vi "ReadDataFromBeckhoff.vi"(6 "error in (no error)":errorcluster, 8 "ReadGrpSymbols":string[](array[string]), 9 "Handle In":u32 format="%x") -> (0 "error out":errorcluster, 1 "BeckhoffParameters":T3, 2 "BeckhoffParamsRawData":T1, 3 "Handle Out":u32)   [LabVIEW 2020]
uses:
  <userlib>/Beckhoff-LabVIEW-Interface/_DependsOn/With TypeResolving/Read Sync Single TypeResolved.vi
panel:
  out "BeckhoffParamReadStatus":T2
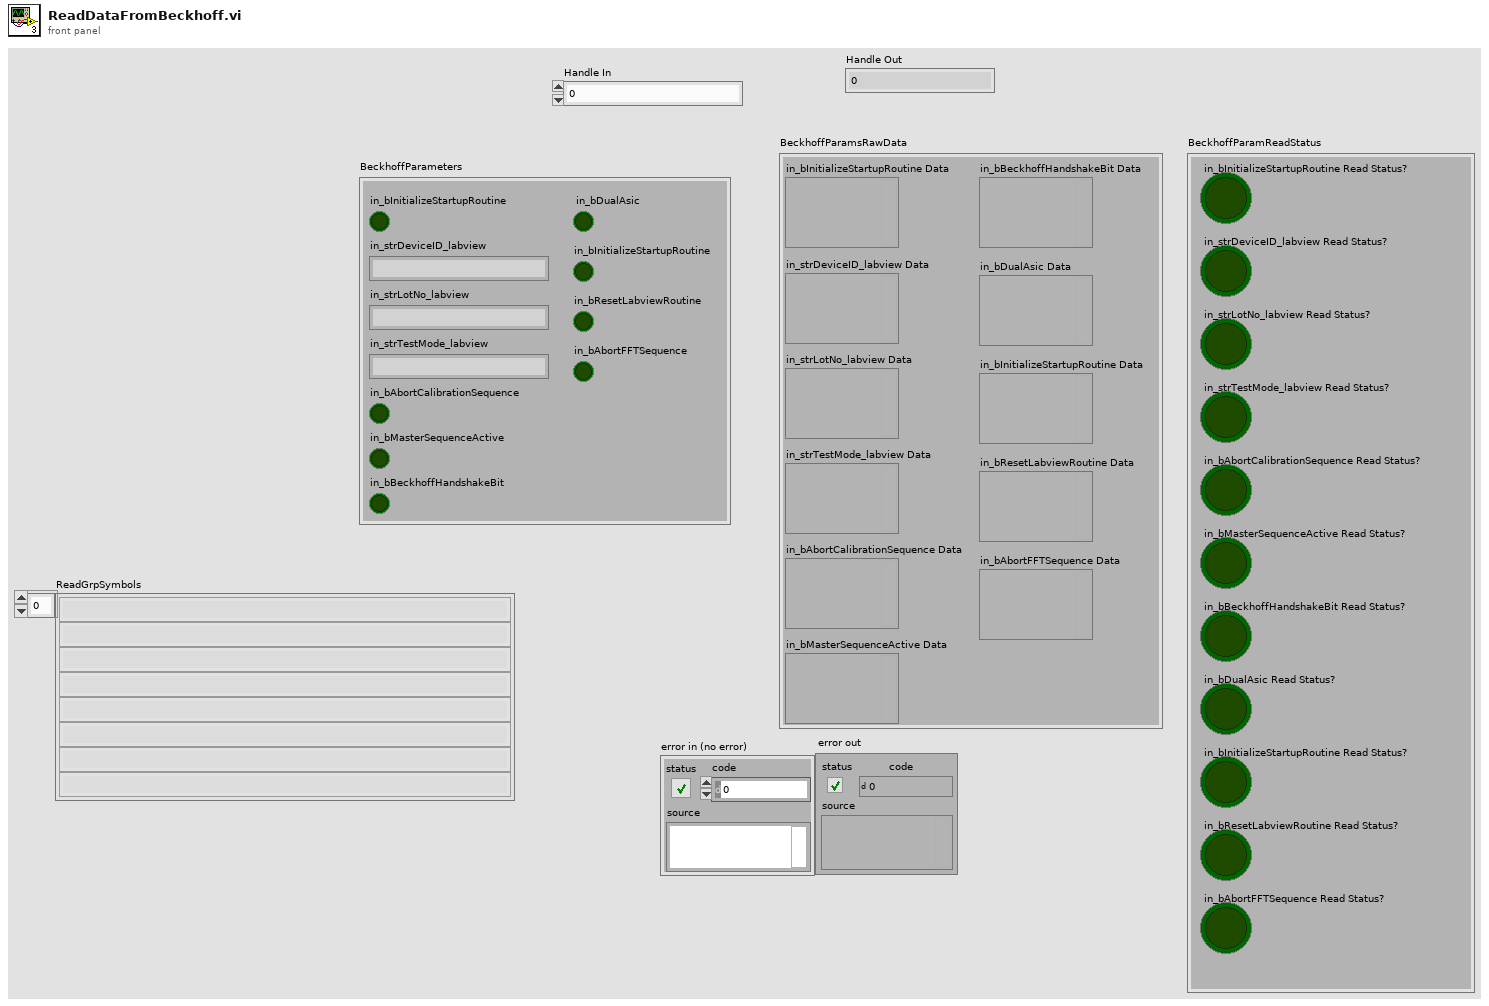
[diagram p1: front panel]
types:
  T1 = cluster{"in_bInitializeStartupRoutine Data":variant, "in_strDeviceID_labview Data":variant, "in_strLotNo_labview Data":variant, "in_strTestMode_labview Data":variant, "in_bAbortCalibrationSequence Data":variant, "in_bMasterSequenceActive Data":variant, "in_bBeckhoffHandshakeBit Data":variant, "in_bDualAsic Data":variant, "in_bInitializeStartupRoutine Data":variant, "in_bResetLabviewRoutine Data":variant, "in_bAbortFFTSequence Data":variant}
  T2 = cluster{"in_bInitializeStartupRoutine Read Status?":bool, "in_strDeviceID_labview Read Status?":bool, "in_strLotNo_labview Read Status?":bool, "in_strTestMode_labview Read Status?":bool, "in_bAbortCalibrationSequence Read Status?":bool, "in_bMasterSequenceActive Read Status?":bool, "in_bBeckhoffHandshakeBit Read Status?":bool, "in_bDualAsic Read Status?":bool, "in_bInitializeStartupRoutine Read Status?":bool, "in_bResetLabviewRoutine Read Status?":bool, "in_bAbortFFTSequence Read Status?":bool}
  T3 = cluster{"in_bInitializeStartupRoutine":bool, "in_strDeviceID_labview":string, "in_strLotNo_labview":string, "in_strTestMode_labview":string, "in_bAbortCalibrationSequence":bool, "in_bMasterSequenceActive":bool, "in_bBeckhoffHandshakeBit":bool, "in_bDualAsic":bool, "in_bInitializeStartupRoutine":bool, "in_bResetLabviewRoutine":bool, "in_bAbortFFTSequence":bool}
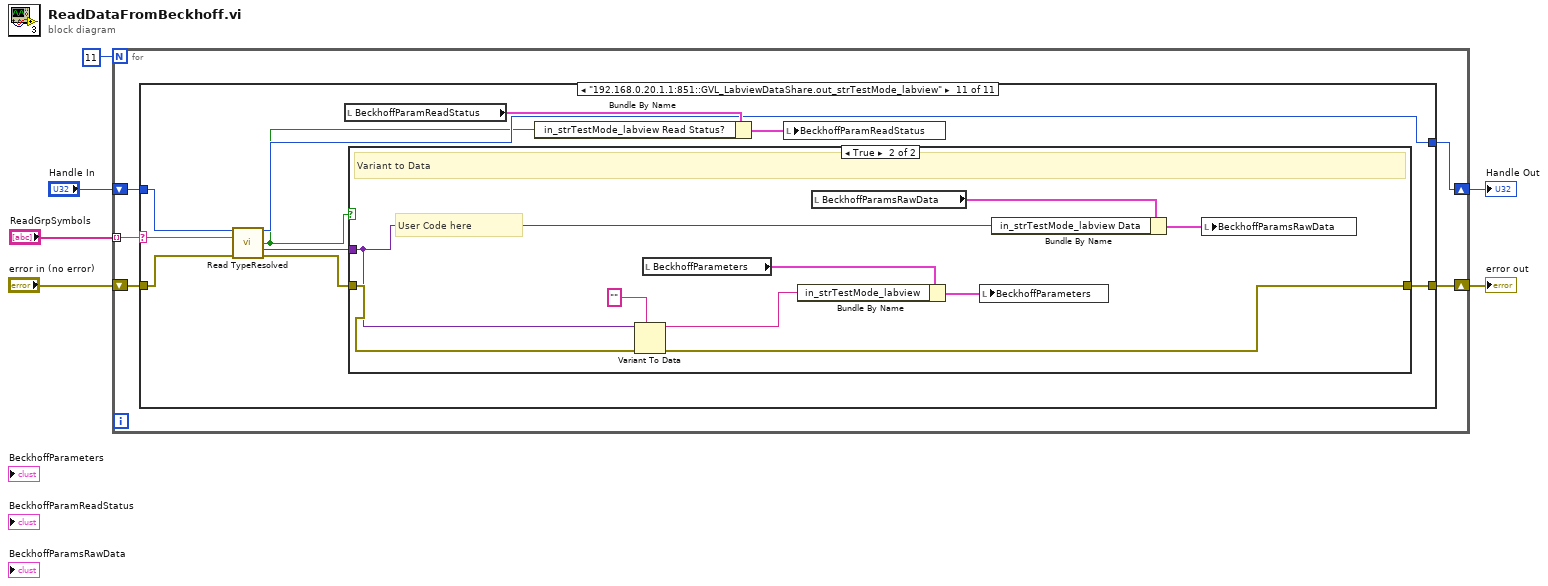
[diagram p0: block diagram]
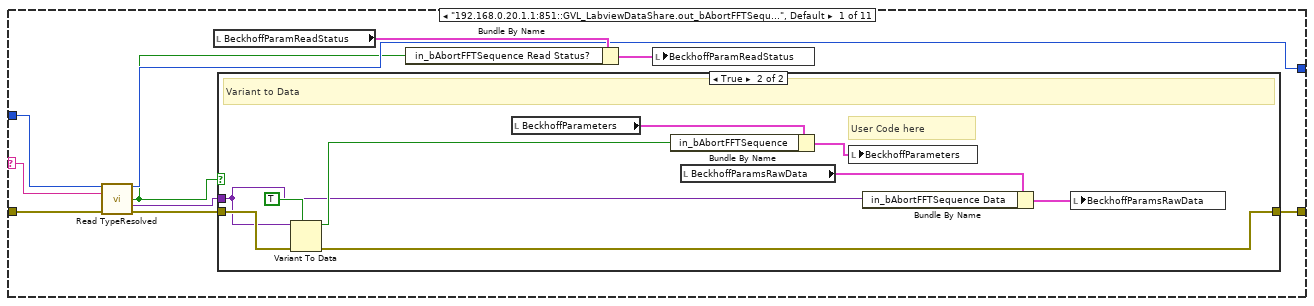
[diagram p2: hidden frame]
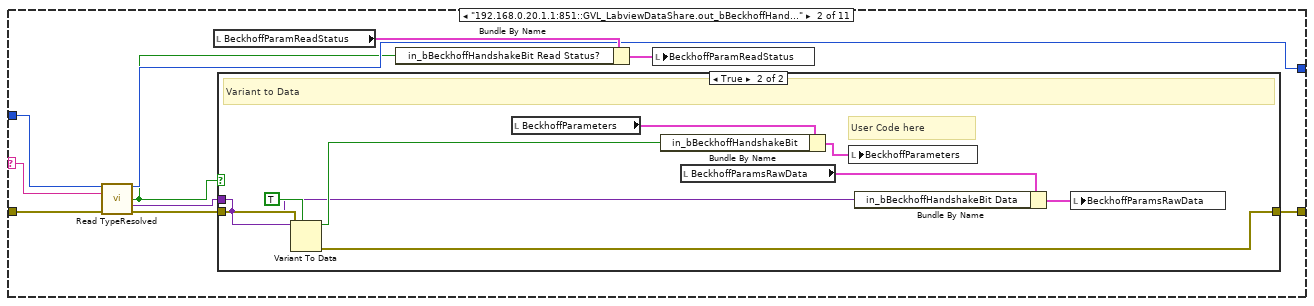
[diagram p4: hidden frame]
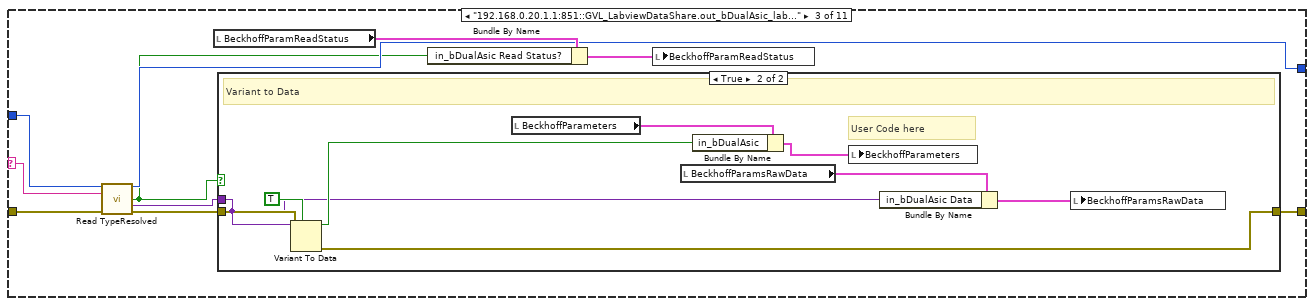
[diagram p6: hidden frame]
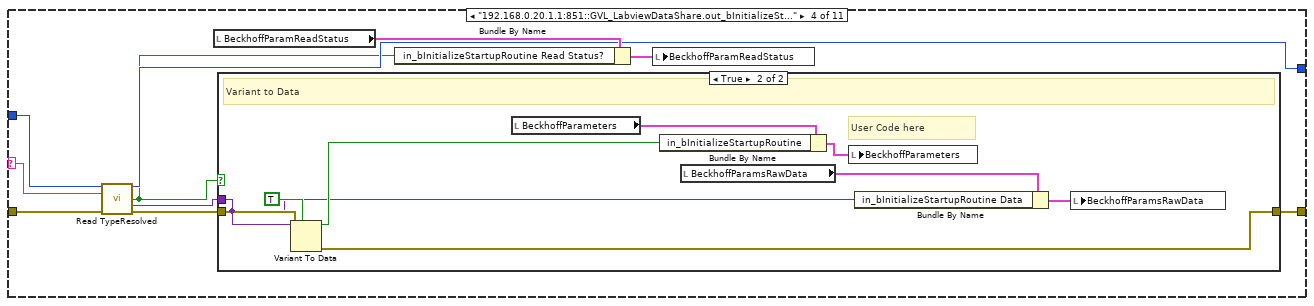
[diagram p8: hidden frame]
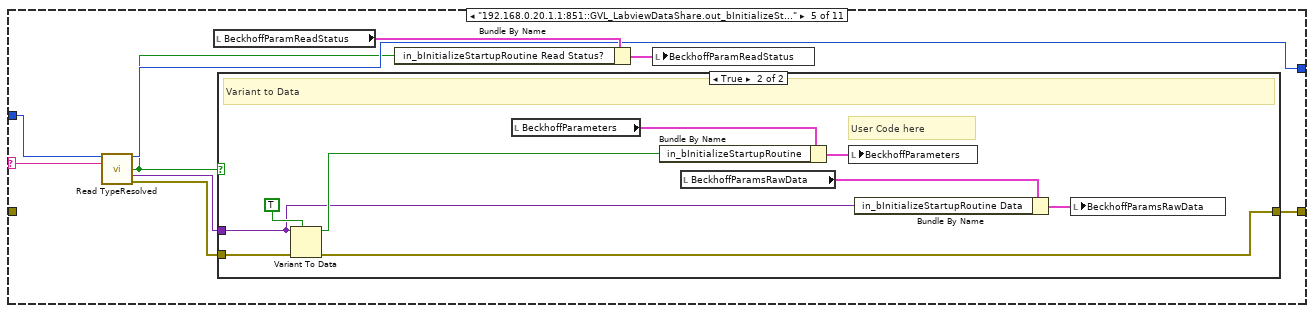
[diagram p10: hidden frame]
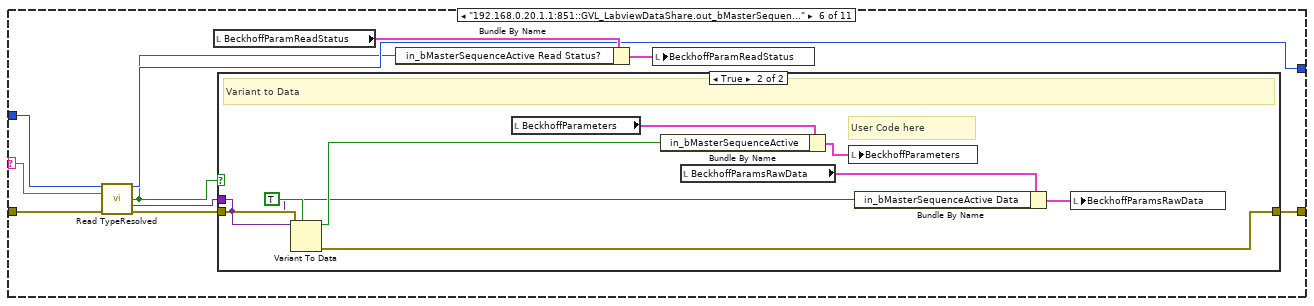
[diagram p12: hidden frame]
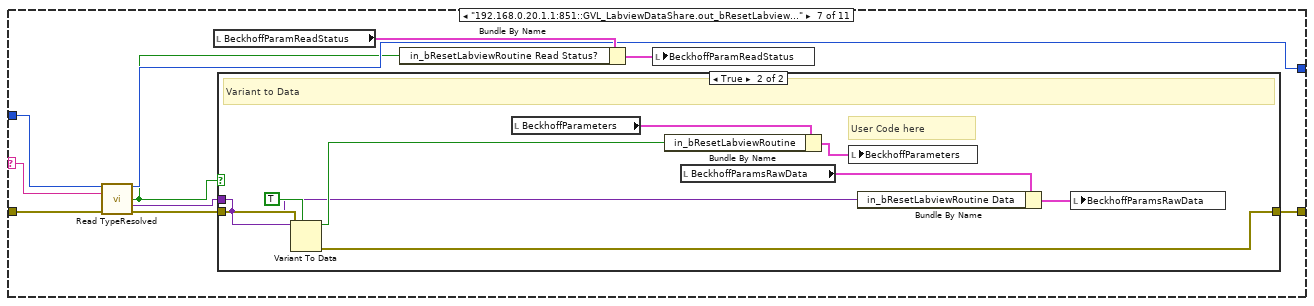
[diagram p14: hidden frame]
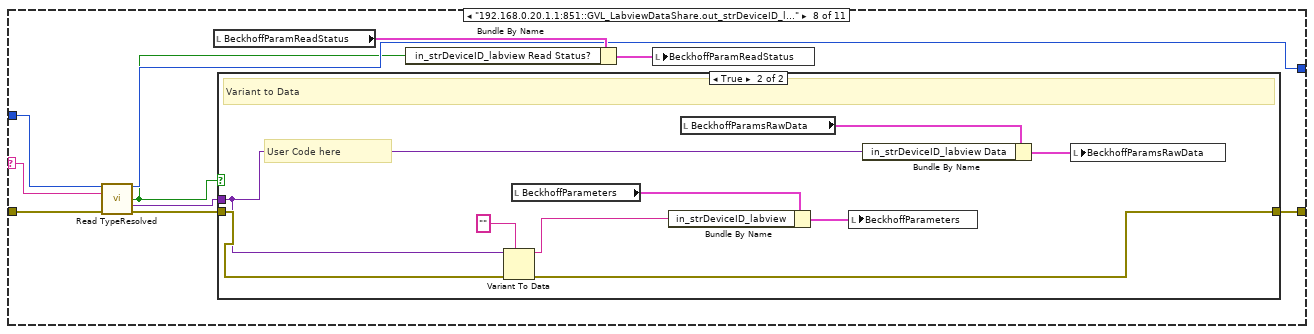
[diagram p16: hidden frame]
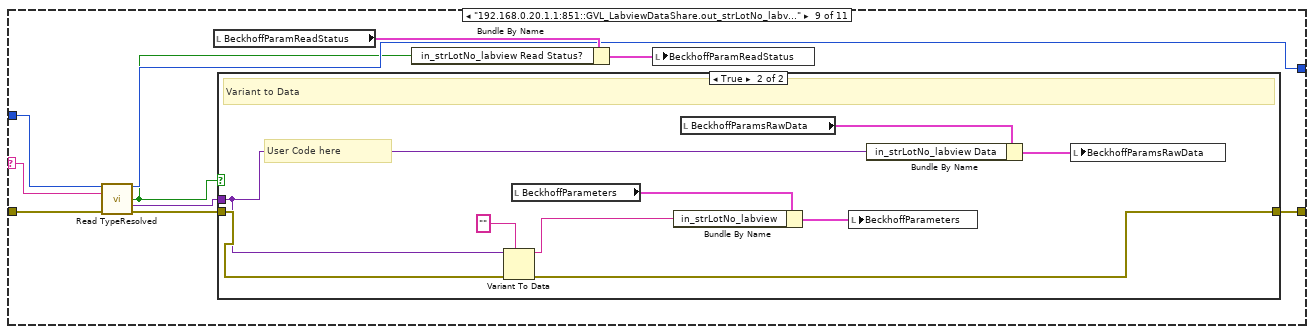
[diagram p18: hidden frame]
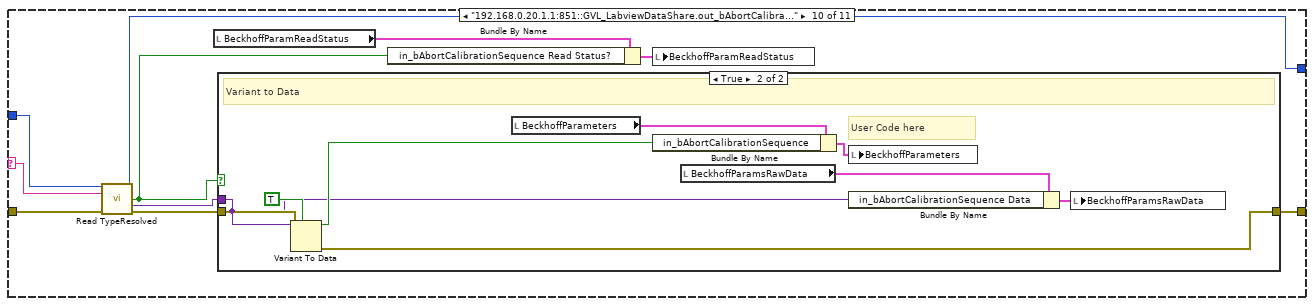
[diagram p20: hidden frame]
diagram:
  n1 = for {
    N: 11 -> [_]
    tunnel: "ReadGrpSymbols" -> [w11] mode=indexing
    shift-right: [w9] -> w2
    shift-left: "error in (no error)" -> [w10]
    shift-right: [w7] -> w1
    shift-left: "Handle In" -> [w8]
    n2 = case shown="\"192.168.0.20.1.1:851::GVL_LabviewDataShare.out_strTestMode_labview\"" w11 {
      selector: w11 -> [w15 w34 w54 w74 w96 w114 w135 w154 w174 w197 w214]
      tunnel: w10 -> [w16 w36 w55 w75 _ w115 w136 w155 w175 w200 w215]
      tunnel: [w13 w37 w57 w77 w93 w116 w132 w156 w176 w193 w216] -> w9
      tunnel: w8 -> [w17 w35 w56 w76 w95 w113 w134 w153 w173 w199 w213]
      tunnel: [w14 w33 w53 w73 w94 w112 w133 w152 w172 w198 w212] -> w7
      frame "192.168.0.20.1.1:851::GVL_LabviewDataShare.out_bAbortFFTSequence_labview", Default {
        n3 = call-poly <userlib>:"Read TypeResolved.vi"("Handle"=w17, "SymbolName"=w15, "error constant"=w16) -> ("Handle"=w14:u32, "Read Status?"=w12:bool, "RData"=w18:variant, "error out"=w19:errorcluster)  [unwired: 9 in]
        n4 = local read "BeckhoffParamReadStatus"() -> (w21:T2)
        n5 = case shown="True" w12 {
          tunnel: w19 -> [w22 w31]
          tunnel: [w22 w30] -> w13
          tunnel: w18 -> [_ w23]
          frame False {
            # "Read Data failed"
            # "Read Status"
          }
          frame True {
            # "User Code here"
            # "Variant to Data"
            n6 = Variant To Data(error in=w31, type=TRUE, Variant=w23) -> (data=w26:bool, error out=w30:errorcluster)
            n7 = local read "BeckhoffParameters"() -> (w28:T3)
            n8 = Bundle By Name(cluster=w28, "in_bAbortFFTSequence"=w26) -> (w27:T3)
            n9 = local read "BeckhoffParamsRawData"() -> (w25:T1)
            n10 = local write "BeckhoffParameters"(w27) -> ()
            n11 = Bundle By Name(cluster=w25, "in_bAbortFFTSequence Data"=w23) -> (w24:T1)
            n12 = local write "BeckhoffParamsRawData"(w24) -> ()
          }
        }
        n13 = Bundle By Name(cluster=w21, "in_bAbortFFTSequence Read Status?"=w12) -> (w20:T2)
        n14 = local write "BeckhoffParamReadStatus"(w20) -> ()
      }
      frame "192.168.0.20.1.1:851::GVL_LabviewDataShare.out_bBeckhoffHandshakeBit_labview" {
        n15 = call-poly <userlib>:"Read TypeResolved.vi"("Handle"=w35, "SymbolName"=w34, "error constant"=w36) -> ("Handle"=w33:u32, "Read Status?"=w32:bool, "RData"=w38:variant, "error out"=w39:errorcluster)  [unwired: 9 in]
        n16 = local read "BeckhoffParamReadStatus"() -> (w41:T2)
        n17 = case shown="True" w32 {
          tunnel: w39 -> [w42 w51]
          tunnel: [w42 w50] -> w37
          tunnel: w38 -> [_ w43]
          frame False {
            # "Read Data failed"
            # "Read Status"
          }
          frame True {
            # "User Code here"
            # "Variant to Data"
            n18 = Variant To Data(error in=w51, type=TRUE, Variant=w43) -> (data=w46:bool, error out=w50:errorcluster)
            n19 = local read "BeckhoffParameters"() -> (w48:T3)
            n20 = Bundle By Name(cluster=w48, "in_bBeckhoffHandshakeBit"=w46) -> (w47:T3)
            n21 = local read "BeckhoffParamsRawData"() -> (w44:T1)
            n22 = local write "BeckhoffParameters"(w47) -> ()
            n23 = Bundle By Name(cluster=w44, "in_bBeckhoffHandshakeBit Data"=w43) -> (w45:T1)
            n24 = local write "BeckhoffParamsRawData"(w45) -> ()
          }
        }
        n25 = Bundle By Name(cluster=w41, "in_bBeckhoffHandshakeBit Read Status?"=w32) -> (w40:T2)
        n26 = local write "BeckhoffParamReadStatus"(w40) -> ()
      }
      frame "192.168.0.20.1.1:851::GVL_LabviewDataShare.out_bDualAsic_labview" {
        n27 = call-poly <userlib>:"Read TypeResolved.vi"("Handle"=w56, "SymbolName"=w54, "error constant"=w55) -> ("Handle"=w53:u32, "Read Status?"=w52:bool, "RData"=w58:variant, "error out"=w59:errorcluster)  [unwired: 9 in]
        n28 = local read "BeckhoffParamReadStatus"() -> (w61:T2)
        n29 = case shown="True" w52 {
          tunnel: w59 -> [w62 w71]
          tunnel: [w62 w70] -> w57
          tunnel: w58 -> [_ w63]
          frame False {
            # "Read Data failed"
            # "Read Status"
          }
          frame True {
            # "User Code here"
            # "Variant to Data"
            n30 = Variant To Data(error in=w71, type=TRUE, Variant=w63) -> (data=w66:bool, error out=w70:errorcluster)
            n31 = local read "BeckhoffParameters"() -> (w68:T3)
            n32 = local read "BeckhoffParamsRawData"() -> (w64:T1)
            n33 = Bundle By Name(cluster=w68, "in_bDualAsic"=w66) -> (w67:T3)
            n34 = local write "BeckhoffParameters"(w67) -> ()
            n35 = Bundle By Name(cluster=w64, "in_bDualAsic Data"=w63) -> (w65:T1)
            n36 = local write "BeckhoffParamsRawData"(w65) -> ()
          }
        }
        n37 = Bundle By Name(cluster=w61, "in_bDualAsic Read Status?"=w52) -> (w60:T2)
        n38 = local write "BeckhoffParamReadStatus"(w60) -> ()
      }
      frame "192.168.0.20.1.1:851::GVL_LabviewDataShare.out_bInitializeStartupRoutine" {
        n39 = call-poly <userlib>:"Read TypeResolved.vi"("Handle"=w76, "SymbolName"=w74, "error constant"=w75) -> ("Handle"=w73:u32, "Read Status?"=w72:bool, "RData"=w78:variant, "error out"=w79:errorcluster)  [unwired: 9 in]
        n40 = local read "BeckhoffParamReadStatus"() -> (w81:T2)
        n41 = case shown="True" w72 {
          tunnel: w79 -> [w82 w91]
          tunnel: [w82 w90] -> w77
          tunnel: w78 -> [_ w83]
          frame False {
            # "Read Data failed"
            # "Read Status"
          }
          frame True {
            # "User Code here"
            # "Variant to Data"
            n42 = Variant To Data(error in=w91, type=TRUE, Variant=w83) -> (data=w86:bool, error out=w90:errorcluster)
            n43 = local read "BeckhoffParameters"() -> (w88:T3)
            n44 = Bundle By Name(cluster=w88, "in_bInitializeStartupRoutine"=w86) -> (w87:T3)
            n45 = local read "BeckhoffParamsRawData"() -> (w84:T1)
            n46 = local write "BeckhoffParameters"(w87) -> ()
            n47 = Bundle By Name(cluster=w84, "in_bInitializeStartupRoutine Data"=w83) -> (w85:T1)
            n48 = local write "BeckhoffParamsRawData"(w85) -> ()
          }
        }
        n49 = Bundle By Name(cluster=w81, "in_bInitializeStartupRoutine Read Status?"=w72) -> (w80:T2)
        n50 = local write "BeckhoffParamReadStatus"(w80) -> ()
      }
      frame "192.168.0.20.1.1:851::GVL_LabviewDataShare.out_bInitializeStartupRoutine_labview" {
        n51 = call-poly <userlib>:"Read TypeResolved.vi"("Handle"=w95, "SymbolName"=w96) -> ("Handle"=w94:u32, "Read Status?"=w92:bool, "RData"=w97:variant, "error out"=w98:errorcluster)  [unwired: 10 in]
        n52 = local read "BeckhoffParamReadStatus"() -> (w100:T2)
        n53 = case shown="True" w92 {
          tunnel: w98 -> [w101 w110]
          tunnel: [w101 w109] -> w93
          tunnel: w97 -> [_ w102]
          frame False {
            # "Read Data failed"
            # "Read Status"
          }
          frame True {
            # "User Code here"
            # "Variant to Data"
            n54 = Variant To Data(error in=w110, type=TRUE, Variant=w102) -> (data=w105:bool, error out=w109:errorcluster)
            n55 = local read "BeckhoffParameters"() -> (w107:T3)
            n56 = Bundle By Name(cluster=w107, "in_bInitializeStartupRoutine"=w105) -> (w106:T3)
            n57 = local read "BeckhoffParamsRawData"() -> (w103:T1)
            n58 = local write "BeckhoffParameters"(w106) -> ()
            n59 = Bundle By Name(cluster=w103, "in_bInitializeStartupRoutine Data"=w102) -> (w104:T1)
            n60 = local write "BeckhoffParamsRawData"(w104) -> ()
          }
        }
        n61 = Bundle By Name(cluster=w100, "in_bInitializeStartupRoutine Read Status?"=w92) -> (w99:T2)
        n62 = local write "BeckhoffParamReadStatus"(w99) -> ()
      }
      frame "192.168.0.20.1.1:851::GVL_LabviewDataShare.out_bMasterSequenceActive_labview" {
        n63 = call-poly <userlib>:"Read TypeResolved.vi"("Handle"=w113, "SymbolName"=w114, "error constant"=w115) -> ("Handle"=w112:u32, "Read Status?"=w111:bool, "RData"=w117:variant, "error out"=w118:errorcluster)  [unwired: 9 in]
        n64 = local read "BeckhoffParamReadStatus"() -> (w120:T2)
        n65 = case shown="True" w111 {
          tunnel: w118 -> [w121 w130]
          tunnel: [w121 w129] -> w116
          tunnel: w117 -> [_ w122]
          frame False {
            # "Read Data failed"
            # "Read Status"
          }
          frame True {
            # "User Code here"
            # "Variant to Data"
            n66 = Variant To Data(error in=w130, type=TRUE, Variant=w122) -> (data=w125:bool, error out=w129:errorcluster)
            n67 = local read "BeckhoffParameters"() -> (w127:T3)
            n68 = Bundle By Name(cluster=w127, "in_bMasterSequenceActive"=w125) -> (w126:T3)
            n69 = local read "BeckhoffParamsRawData"() -> (w123:T1)
            n70 = local write "BeckhoffParameters"(w126) -> ()
            n71 = Bundle By Name(cluster=w123, "in_bMasterSequenceActive Data"=w122) -> (w124:T1)
            n72 = local write "BeckhoffParamsRawData"(w124) -> ()
          }
        }
        n73 = Bundle By Name(cluster=w120, "in_bMasterSequenceActive Read Status?"=w111) -> (w119:T2)
        n74 = local write "BeckhoffParamReadStatus"(w119) -> ()
      }
      frame "192.168.0.20.1.1:851::GVL_LabviewDataShare.out_bResetLabviewRoutine_labview" {
        n75 = call-poly <userlib>:"Read TypeResolved.vi"("Handle"=w134, "SymbolName"=w135, "error constant"=w136) -> ("Handle"=w133:u32, "Read Status?"=w131:bool, "RData"=w137:variant, "error out"=w138:errorcluster)  [unwired: 9 in]
        n76 = local read "BeckhoffParamReadStatus"() -> (w140:T2)
        n77 = case shown="True" w131 {
          tunnel: w138 -> [w141 w150]
          tunnel: [w141 w149] -> w132
          tunnel: w137 -> [_ w142]
          frame False {
            # "Read Data failed"
            # "Read Status"
          }
          frame True {
            # "User Code here"
            # "Variant to Data"
            n78 = Variant To Data(error in=w150, type=TRUE, Variant=w142) -> (data=w145:bool, error out=w149:errorcluster)
            n79 = local read "BeckhoffParameters"() -> (w147:T3)
            n80 = Bundle By Name(cluster=w147, "in_bResetLabviewRoutine"=w145) -> (w146:T3)
            n81 = local read "BeckhoffParamsRawData"() -> (w144:T1)
            n82 = local write "BeckhoffParameters"(w146) -> ()
            n83 = Bundle By Name(cluster=w144, "in_bResetLabviewRoutine Data"=w142) -> (w143:T1)
            n84 = local write "BeckhoffParamsRawData"(w143) -> ()
          }
        }
        n85 = Bundle By Name(cluster=w140, "in_bResetLabviewRoutine Read Status?"=w131) -> (w139:T2)
        n86 = local write "BeckhoffParamReadStatus"(w139) -> ()
      }
      frame "192.168.0.20.1.1:851::GVL_LabviewDataShare.out_strDeviceID_labview" {
        n87 = call-poly <userlib>:"Read TypeResolved.vi"("Handle"=w153, "SymbolName"=w154, "error constant"=w155) -> ("Handle"=w152:u32, "Read Status?"=w151:bool, "RData"=w157:variant, "error out"=w158:errorcluster)  [unwired: 9 in]
        n88 = local read "BeckhoffParamReadStatus"() -> (w160:T2)
        n89 = case shown="True" w151 {
          tunnel: w158 -> [w161 w170]
          tunnel: [w161 w169] -> w156
          tunnel: w157 -> [_ w162]
          frame False {
            # "Read Data failed"
            # "Read Status"
          }
          frame True {
            # "User Code here"
            # "Variant to Data"
            n90 = Variant To Data(error in=w170, type="", Variant=w162) -> (data=w165:string, error out=w169:errorcluster)
            n91 = local read "BeckhoffParameters"() -> (w167:T3)
            n92 = Bundle By Name(cluster=w167, "in_strDeviceID_labview"=w165) -> (w166:T3)
            n93 = local read "BeckhoffParamsRawData"() -> (w164:T1)
            n94 = local write "BeckhoffParameters"(w166) -> ()
            n95 = Bundle By Name(cluster=w164, "in_strDeviceID_labview Data"=w162) -> (w163:T1)
            n96 = local write "BeckhoffParamsRawData"(w163) -> ()
          }
        }
        n97 = Bundle By Name(cluster=w160, "in_strDeviceID_labview Read Status?"=w151) -> (w159:T2)
        n98 = local write "BeckhoffParamReadStatus"(w159) -> ()
      }
      frame "192.168.0.20.1.1:851::GVL_LabviewDataShare.out_strLotNo_labview" {
        n99 = call-poly <userlib>:"Read TypeResolved.vi"("Handle"=w173, "SymbolName"=w174, "error constant"=w175) -> ("Handle"=w172:u32, "Read Status?"=w171:bool, "RData"=w177:variant, "error out"=w178:errorcluster)  [unwired: 9 in]
        n100 = local read "BeckhoffParamReadStatus"() -> (w180:T2)
        n101 = case shown="True" w171 {
          tunnel: w178 -> [w181 w190]
          tunnel: [w181 w189] -> w176
          tunnel: w177 -> [_ w182]
          frame False {
            # "Read Data failed"
            # "Read Status"
          }
          frame True {
            # "User Code here"
            # "Variant to Data"
            n102 = Variant To Data(error in=w190, type="", Variant=w182) -> (data=w185:string, error out=w189:errorcluster)
            n103 = local read "BeckhoffParameters"() -> (w187:T3)
            n104 = Bundle By Name(cluster=w187, "in_strLotNo_labview"=w185) -> (w186:T3)
            n105 = local read "BeckhoffParamsRawData"() -> (w183:T1)
            n106 = local write "BeckhoffParameters"(w186) -> ()
            n107 = Bundle By Name(cluster=w183, "in_strLotNo_labview Data"=w182) -> (w184:T1)
            n108 = local write "BeckhoffParamsRawData"(w184) -> ()
          }
        }
        n109 = Bundle By Name(cluster=w180, "in_strLotNo_labview Read Status?"=w171) -> (w179:T2)
        n110 = local write "BeckhoffParamReadStatus"(w179) -> ()
      }
      frame "192.168.0.20.1.1:851::GVL_LabviewDataShare.out_bAbortCalibrationSequence_labview" {
        n111 = call-poly <userlib>:"Read TypeResolved.vi"("Handle"=w199, "SymbolName"=w197, "error constant"=w200) -> ("Handle"=w198:u32, "Read Status?"=w191:bool, "RData"=w192:variant, "error out"=w194:errorcluster)  [unwired: 9 in]
        n112 = local read "BeckhoffParamReadStatus"() -> (w196:T2)
        n113 = case shown="True" w191 {
          tunnel: w194 -> [w201 w210]
          tunnel: [w201 w209] -> w193
          tunnel: w192 -> [_ w202]
          frame False {
            # "Read Data failed"
            # "Read Status"
          }
          frame True {
            # "User Code here"
            # "Variant to Data"
            n114 = Variant To Data(error in=w210, type=TRUE, Variant=w202) -> (data=w205:bool, error out=w209:errorcluster)
            n115 = local read "BeckhoffParameters"() -> (w207:T3)
            n116 = Bundle By Name(cluster=w207, "in_bAbortCalibrationSequence"=w205) -> (w206:T3)
            n117 = local read "BeckhoffParamsRawData"() -> (w203:T1)
            n118 = local write "BeckhoffParameters"(w206) -> ()
            n119 = Bundle By Name(cluster=w203, "in_bAbortCalibrationSequence Data"=w202) -> (w204:T1)
            n120 = local write "BeckhoffParamsRawData"(w204) -> ()
          }
        }
        n121 = Bundle By Name(cluster=w196, "in_bAbortCalibrationSequence Read Status?"=w191) -> (w195:T2)
        n122 = local write "BeckhoffParamReadStatus"(w195) -> ()
      }
      frame "192.168.0.20.1.1:851::GVL_LabviewDataShare.out_strTestMode_labview" {
        n123 = call-poly <userlib>:"Read TypeResolved.vi"("Handle"=w213, "SymbolName"=w214, "error constant"=w215) -> ("Handle"=w212:u32, "Read Status?"=w211:bool, "RData"=w217:variant, "error out"=w218:errorcluster)  [unwired: 9 in]
        n124 = local read "BeckhoffParamReadStatus"() -> (w220:T2)
        n125 = case shown="True" w211 {
          tunnel: w218 -> [w221 w230]
          tunnel: [w221 w229] -> w216
          tunnel: w217 -> [_ w222]
          frame False {
            # "Read Data failed"
            # "Read Status"
          }
          frame True {
            # "User Code here"
            # "Variant to Data"
            n126 = Variant To Data(error in=w230, type="", Variant=w222) -> (data=w225:string, error out=w229:errorcluster)
            n127 = local read "BeckhoffParameters"() -> (w227:T3)
            n128 = Bundle By Name(cluster=w227, "in_strTestMode_labview"=w225) -> (w226:T3)
            n129 = local read "BeckhoffParamsRawData"() -> (w224:T1)
            n130 = local write "BeckhoffParameters"(w226) -> ()
            n131 = Bundle By Name(cluster=w224, "in_strTestMode_labview Data"=w222) -> (w223:T1)
            n132 = local write "BeckhoffParamsRawData"(w223) -> ()
          }
        }
        n133 = Bundle By Name(cluster=w220, "in_strTestMode_labview Read Status?"=w211) -> (w219:T2)
        n134 = local write "BeckhoffParamReadStatus"(w219) -> ()
      }
    }
  }
  "error out" <- w2
  "Handle Out" <- w1
